vi "ArcadeJoystick.vi"(6 "Max Output":dbl=1.0, 7 "Square Inputs":bool=TRUE, 9 "Y axis value":dbl, 10 "X axis value":dbl) -> (1 "Right Motor Value":dbl, 2 "Left Motor Value":dbl)   [LabVIEW 2019]
doc: "Uses a standard algorithm to map joystick axes into motor updates for arcade driving. This algorithm does not saturate over half of the range.\n\nThis software is licensed. Open the labview\\readme\\WPI Robotics Library Open Source License.txt file for more information."
panel:
  in  "Turning Sensitivity":dbl=1.0
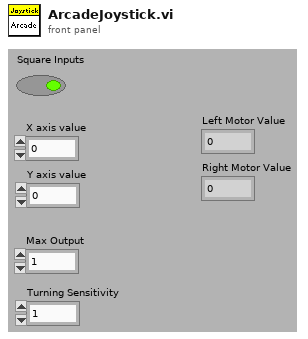
[diagram p1: front panel]
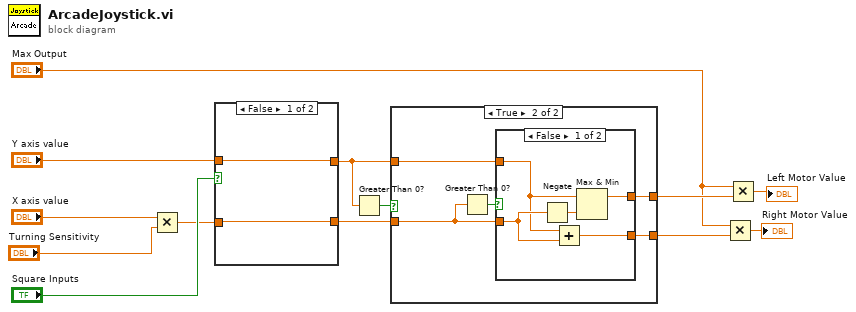
[diagram p0: block diagram]
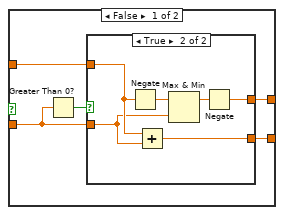
[diagram p2: hidden frame]
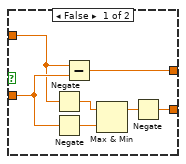
[diagram p3: hidden frame]
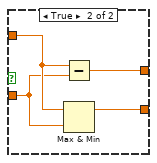
[diagram p4: hidden frame]
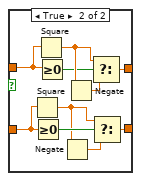
[diagram p5: hidden frame]
diagram:
  n1 = Multiply(x="X axis value", y="Turning Sensitivity") -> (x*y=w2:dbl)
  n2 = case shown="False" "Square Inputs" {
    tunnel: [w14 w25] -> w11
    tunnel: [w15 w24] -> w12
    tunnel: w2 -> [w14 w23]
    tunnel: "Y axis value" -> [w15 w22]
    frame False {
    }
    frame True {
      n3 = Square(x=w23) -> (x^2=w20:dbl)
      n4 = Greater Or Equal To 0?(x=w23) -> (x >= 0?=w21:bool)
      n5 = Square(x=w22) -> (x^2=w17:dbl)
      n6 = Greater Or Equal To 0?(x=w22) -> (x >= 0?=w16:bool)
      n7 = Negate(x=w20) -> (-x=w19:dbl)
      n8 = Negate(x=w17) -> (-x=w18:dbl)
      n9 = Select(t=w17, s=w16, f=w18) -> (s? t:f=w24:dbl)
      n10 = Select(t=w20, s=w21, f=w19) -> (s? t:f=w25:dbl)
    }
  }
  n11 = Greater Than 0?(x=w12) -> (x > 0?=w13:bool)
  n12 = case shown="True" w13 {
    tunnel: w11 -> [w29 w47]
    tunnel: w12 -> [w28 w46]
    tunnel: [w27 w45] -> w10
    tunnel: [w26 w44] -> w8
    frame False {
      n13 = Greater Than 0?(x=w29) -> (x > 0?=w30:bool)
      n14 = case shown="True" w30 {
        tunnel: w29 -> [w37 w39]
        tunnel: w28 -> [w35 w40]
        tunnel: [w31 w41] -> w27
        tunnel: [w32 w38] -> w26
        frame False {
          n15 = Negate(x=w35) -> (-x=w36:dbl)
          n16 = Negate(x=w37) -> (-x=w34:dbl)
          n17 = Subtract(x=w35, y=w37) -> (x-y=w31:dbl)
          n18 = Max & Min(x=w36, y=w34) -> (max(x,y)=w33:dbl)  [unwired: 1 out]
          n19 = Negate(x=w33) -> (-x=w32:dbl)
        }
        frame True {
          n20 = Negate(x=w40) -> (-x=w43:dbl)
          n21 = Add(x=w40, y=w39) -> (x+y=w38:dbl)
          n22 = Max & Min(x=w43, y=w39) -> (max(x,y)=w42:dbl)  [unwired: 1 out]
          n23 = Negate(x=w42) -> (-x=w41:dbl)
        }
      }
    }
    frame True {
      n24 = Greater Than 0?(x=w47) -> (x > 0?=w48:bool)
      n25 = case shown="False" w48 {
        tunnel: w47 -> [w53 w55]
        tunnel: w46 -> [w50 w56]
        tunnel: [w51 w54] -> w45
        tunnel: [w49 w57] -> w44
        frame False {
          n26 = Negate(x=w53) -> (-x=w52:dbl)
          n27 = Add(x=w50, y=w53) -> (x+y=w49:dbl)
          n28 = Max & Min(x=w50, y=w52) -> (max(x,y)=w51:dbl)  [unwired: 1 out]
        }
        frame True {
          n29 = Subtract(x=w56, y=w55) -> (x-y=w54:dbl)
          n30 = Max & Min(x=w56, y=w55) -> (max(x,y)=w57:dbl)  [unwired: 1 out]
        }
      }
    }
  }
  n31 = Multiply(x="Max Output", y=w8) -> (x*y=→"Right Motor Value":dbl)
  n32 = Multiply(x="Max Output", y=w10) -> (x*y=→"Left Motor Value":dbl)
